vi "Initialise.vi"(7 "Initial DI":T1, 8 "error in (no error)":errorcluster, 9 "Robot Frame":string, 10 "Robot Name":string, 11 "Master in":refnum<class "GripsMaster.lvclass">) -> (0 "error out":errorcluster, 3 "Master out":refnum<class "GripsMaster.lvclass">)   [LabVIEW 2011, in "GripsMaster.lvclass"]
uses:
  GripsMaster.lvclass
  Controls/Digital Values.ctl
  Controls/Analog Values.ctl
  GripsMaster.lvclass/GripsMaster.ctl
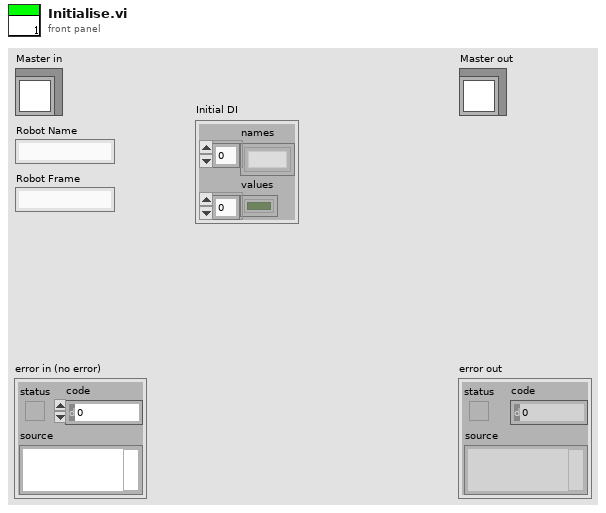
[diagram p1: front panel]
types:
  T1 = typedef "Digital Values.ctl" = cluster{"names":string[], "values":bool[]}
  T2 = typedef "Analog Values.ctl" = cluster{"names":string[], "values":dbl[]}
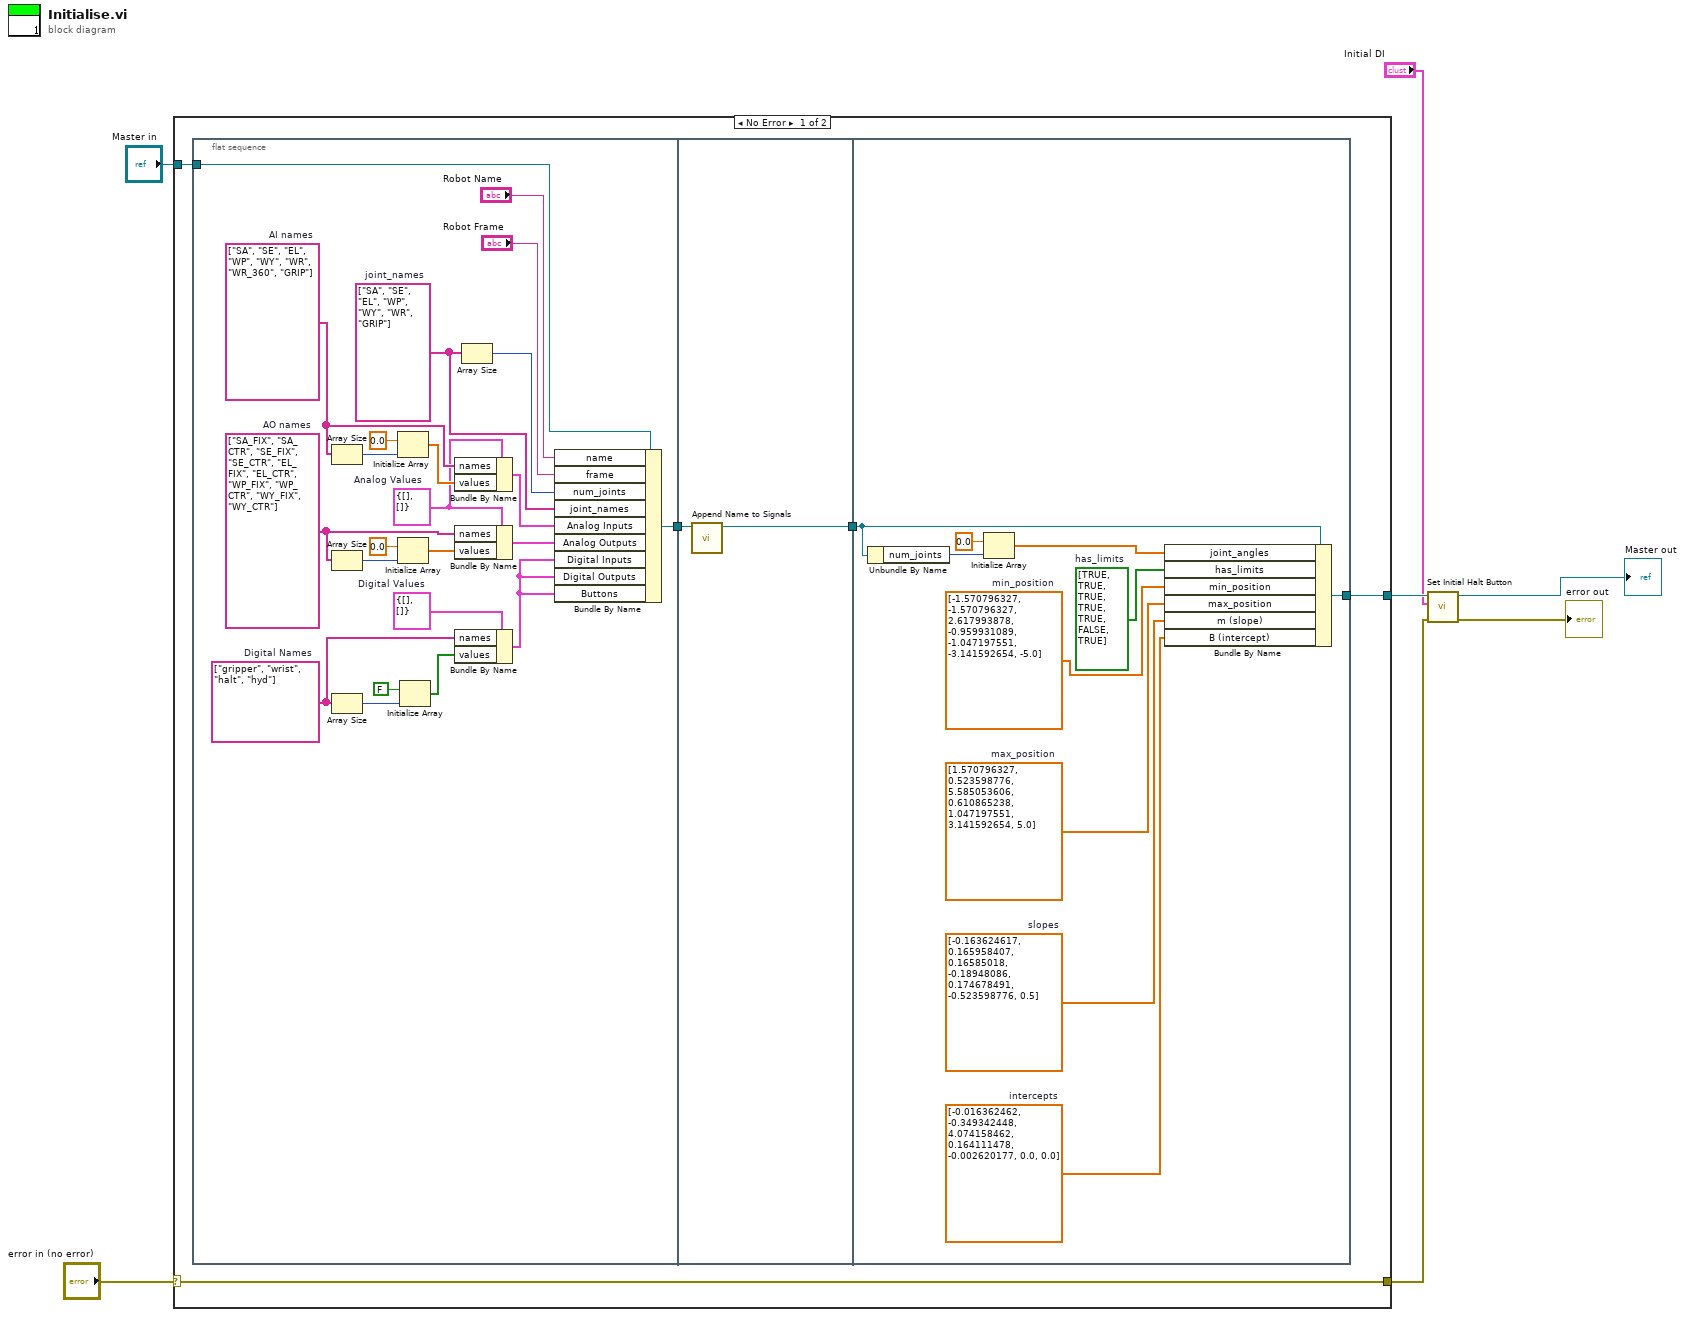
[diagram p0: block diagram]
diagram:
  n1 = case shown="No Error" "error in (no error)" {
    selector: "error in (no error)" -> [w8 w49]
    tunnel: [w8 w49] -> w4
    tunnel: [w10 w48] -> w5
    tunnel: "Master in" -> [w12 w48]
    frame No Error {
      n2 = flat-sequence {
        tunnel: w12 -> [w35]
        tunnel: [w13] -> w11
        tunnel: w11 -> [w37]
        tunnel: [w36] -> w9
        tunnel: [w47] -> w10
        tunnel: w9 -> [w41]
        frame #0 {
          w23 = T2 {"names"=[], "values"=[]}  # Analog Values
          w19 = string[] ["gripper", "wrist", "halt", "hyd"]  # Digital Names
          w31 = string[] ["SA_FIX", "SA_CTR", "SE_FIX", "SE_CTR", "EL_FIX", "EL_CTR", "WP_FIX", "WP_CTR", "WY_FIX", "WY_CTR"]  # AO names
          w28 = string[] ["SA", "SE", "EL", "WP", "WY", "WR", "WR_360", "GRIP"]  # AI names
          w21 = T1 {"names"=[], "values"=[]}  # Digital Values
          w16 = string[] ["SA", "SE", "EL", "WP", "WY", "WR", "GRIP"]  # joint_names
          n3 = Array Size(array=w28) -> (size(s)=w27:i32)
          n4 = Array Size(array=w31) -> (size(s)=w30:i32)
          n5 = Array Size(array=w19) -> (size(s)=w20:i32)
          n6 = Initialize Array(0.0 ("element"), w27) -> (w25:dbl[])
          n7 = Initialize Array(0.0 ("element"), w30) -> (w29:dbl[])
          n8 = Initialize Array(FALSE, w20) -> (w18:bool[])
          n9 = Bundle By Name(cluster=w23, "names"=w28, "values"=w25) -> (w24:T2)
          n10 = Bundle By Name(cluster=w23, "names"=w31, "values"=w29) -> (w22:T2)
          n11 = Bundle By Name(cluster=w21, "names"=w19, "values"=w18) -> (w14:T1)
          n12 = Array Size(array=w16) -> (size(s)=w15:i32)
          n13 = Bundle By Name(cluster=w35, "name"="Robot Name", "frame"="Robot Frame", "num_joints"=w15, "joint_names"=w16, "Analog Inputs"=w24, "Analog Outputs"=w22, "Digital Inputs"=w14, "Digital Outputs"=w14, "Buttons"=w14) -> (w13:refnum<class "GripsMaster.lvclass">)
        }
        frame #1 {
          n14 = call "Append Name to Signals.vi"("GripsMaster in"=w37) -> ("GripsMaster out"=w36:refnum<class "GripsMaster.lvclass">)  [unwired: 9 in, 1 out]
        }
        frame #2 {
          w42 = dbl[] [-0.016362462, -0.349342448, 4.074158462, 0.164111478, -0.002620177, 0.0, 0.0]  # intercepts
          w43 = dbl[] [-0.163624617, 0.165958407, 0.16585018, -0.18948086, 0.174678491, -0.523598776, 0.5]  # slopes
          w44 = dbl[] [-1.570796327, -1.570796327, 2.617993878, -0.959931089, -1.047197551, -3.141592654, -5.0]  # min_position
          w45 = dbl[] [1.570796327, 0.523598776, 5.585053606, 0.610865238, 1.047197551, 3.141592654, 5.0]  # max_position
          w46 = bool[] [TRUE, TRUE, TRUE, TRUE, TRUE, FALSE, TRUE]  # has_limits
          n15 = Unbundle By Name(w41) -> ("num_joints"=w39:i32)
          n16 = Initialize Array(0.0 ("element"), w39) -> (w38:dbl[])
          n17 = Bundle By Name(cluster=w41, "joint_angles"=w38, "has_limits"=w46, "min_position"=w44, "max_position"=w45, "m (slope)"=w43, "B (intercept)"=w42) -> (w47:refnum<class "GripsMaster.lvclass">)
        }
      }
    }
    frame Error {
    }
  }
  n18 = call "Set Initial Halt Button.vi"("error in (no error)"=w4, "Digital Inputs"="Initial DI", "GripsMaster in"=w5) -> ("error out"=→"error out":errorcluster, "GripsMaster out"=→"Master out":refnum<class "GripsMaster.lvclass">)  [unwired: 7 in]
